vi "k_means.vi"(6 "# máximo de iterações":i32, 8 "altura (pixels)":i32, 9 "largura (pixels)":i32, 10 "K":u16, 11 "point array":cluster{"x":dbl, "y":dbl}[](array[cluster])) -> (3 "Array":T1(array[cluster]))   [LabVIEW 2016]
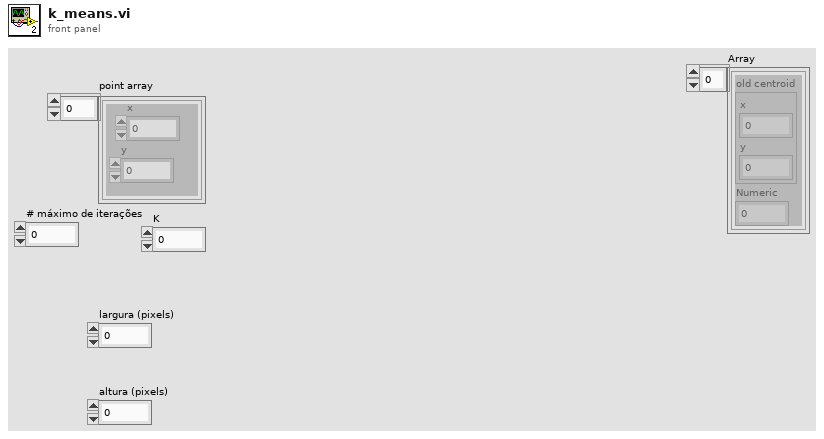
[diagram p1: front panel]
types:
  T1 = cluster{"old centroid":cluster{"x":dbl, "y":dbl}, "Numeric":i32}[]
  T2 = cluster{"point":cluster{"x":dbl, "y":dbl}, "Numeric":i32}
  T3 = cluster{"point":cluster{"x":dbl, "y":dbl}, "centroid out":cluster{"point":cluster{"x":dbl, "y":dbl}, "Numeric":i32}}
  T4 = cluster{"old centroid":cluster{"x":dbl, "y":dbl}, "Numeric":i32}
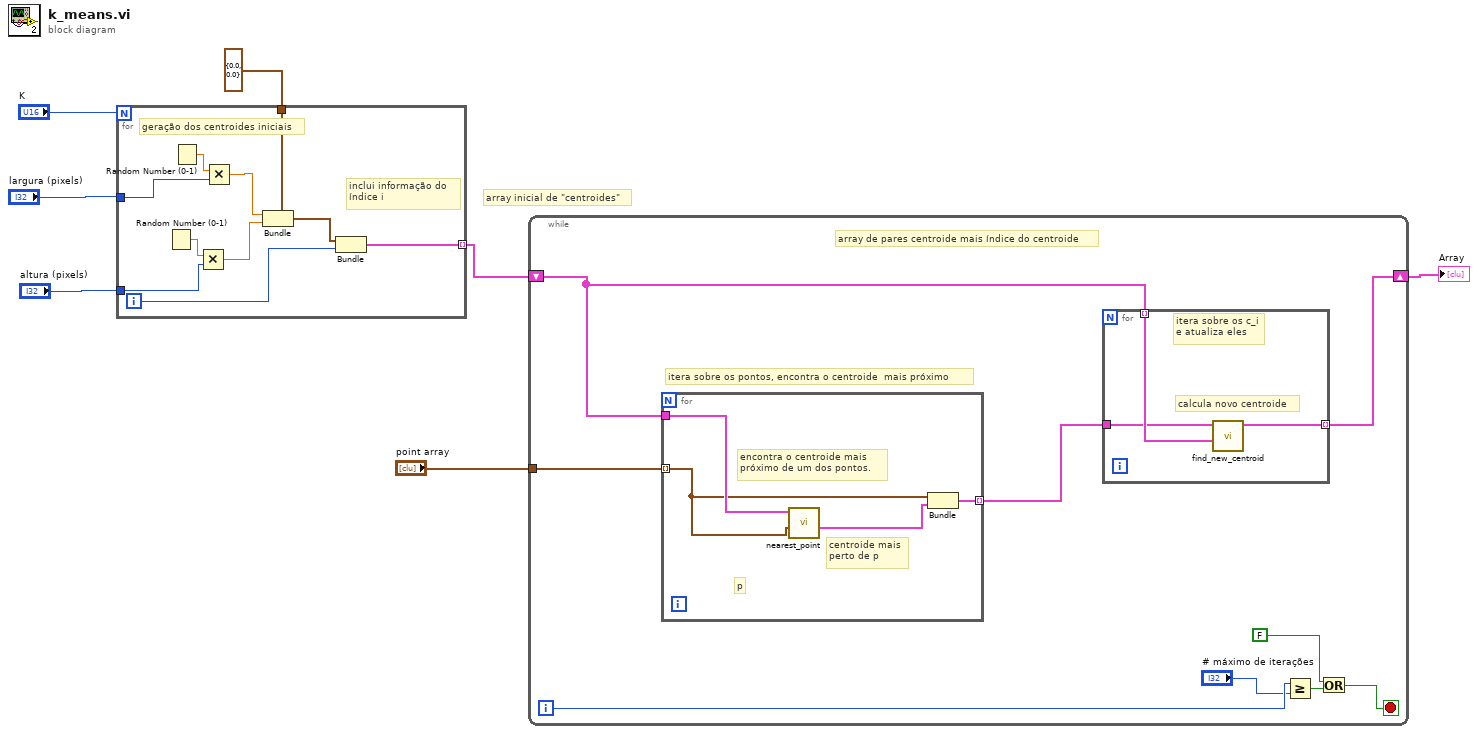
[diagram p0: block diagram]
diagram:
  # "array inicial de \"centroides\""
  n1 = for {
    N: "K" -> [_]
    tunnel: "altura (pixels)" -> [w14]
    tunnel: "largura (pixels)" -> [w15]
    tunnel: cluster{"x":dbl, "y":dbl} {"x"=0.0, "y"=0.0} ("point") -> [w13]
    tunnel: [w9] -> w4 mode=indexing
    i -> [w10]
    # "inclui informação do\níndice i"
    # "geração dos centroides iniciais"
    n2 = Random Number (0-1)() -> (number: 0 to 1=w16:dbl)
    n3 = Random Number (0-1)() -> (number: 0 to 1=w17:dbl)
    n4 = Multiply(x=w16, y=w14) -> (x*y=w11:dbl)
    n5 = Multiply(x=w17, y=w15) -> (x*y=w12:dbl)
    n6 = Bundle(cluster=w13, "x"=w12, "y"=w11) -> (w8:cluster{"x":dbl, "y":dbl})
    n7 = Bundle("point"=w8, w10) -> (w9:cluster{"point":cluster{"x":dbl, "y":dbl}, i32})  [unwired: 1 in]
  }
  n8 = while {
    tunnel: "point array" -> [w26]
    shift-right: [w24] -> w3
    shift-left: w4 -> [w23]
    i -> [w20]
    stop <- w22 stop-if-true
    # "itera sobre os pontos, encontra o centroide  mais próximo"
    # "array de pares centroide mais índice do centroide"
    n9 = for {
      tunnel: w26 -> [w27] mode=indexing
      tunnel: w23 -> [w28]
      tunnel: [w29] -> w25 mode=indexing
      # "centroide mais\nperto de p"
      # "p"
      # "encontra o centroide mais\npróximo de um dos pontos."
      n10 = call "nearest_point.vi"("point in"=w27, "Array in"=w28) -> ("centroid out"=w30:T2)  [unwired: 8 in, 1 out]
      n11 = Bundle("point"=w27, "centroid out"=w30) -> (w29:T3)  [unwired: 1 in]
    }
    n12 = for {
      tunnel: w23 -> [w33] mode=indexing
      tunnel: w25 -> [w32]
      tunnel: [w31] -> w24 mode=indexing
      # "calcula novo centroide"
      # "itera sobre os c_i\ne atualiza eles"
      n13 = call "find_new_centroid.vi"("centroide (ponto, índice)"=w33, "Array"=w32) -> ("centroide (ponto, índice) 2"=w31:T4)  [unwired: 9 in]
    }
    n14 = Greater Or Equal?(x=w20, y="# máximo de iterações") -> (x >= y?=w21:bool)
    n15 = Or(x=FALSE ("y"), y=w21) -> (x .or. y?=w22:bool)
  }
  "Array" <- w3
